vi "test_RxUDPBlockRead.vi"() -> ()   [LabVIEW 2020]
uses:
  <instrlib>/AIM GmbH/_AIM 664/_controls/comm_computedMAC-IP.ctl
  <instrlib>/AIM GmbH/_AIM 664/_controls/comm_verification_rx.ctl
  <instrlib>/AIM GmbH/_AIM 664/_controls/comm_udp_rx.ctl
  <instrlib>/AIM GmbH/_AIM 664/bsp/Controls/ReceiveUDPBlockRead.ctl
  <instrlib>/AIM GmbH/_AIM 664/bsp/Fdx Create Session (Rx-VL-Oriented).vi
  <instrlib>/AIM GmbH/_AIM 664/bsp/Receive/FdxCreateRxVL.vi
  <instrlib>/AIM GmbH/_AIM 664/bsp/Fdx Create UDP Port (RX-CommPort).vi
  <instrlib>/AIM GmbH/_AIM 664/bsp/Fdx Start (Rx).vi
  <instrlib>/AIM GmbH/_AIM 664/bsp/Fdx Stop (Rx).vi
  <instrlib>/AIM GmbH/_AIM 664/AIM664LV.lvlib
panel:
  out "size(s)":i32
  out "RxUDPBlockReadInPortArray":T1[](array[typedef]) {"UDP Handle Out" format="%.0x"; "UDP Handle" format="%.0x"; "Message Buffer" format="%.0x"}
  out "read time uS":u32(graph)
  out "MsgRead Total":u32
  in  "rx fetch rate mS":u32=100
  out "GlobalStat Out":T2={"TotalByteCount"=[139198, 0, 0, 0, 0, 0, 0, 0], "FrameGoodCount"=[1762, 0, 0, 0, 0, 0, 0, 0], "FrameErrorCount"=[0, 0, 0, 0, 0, 0, 0, 0], "BytesPerSecond"=[15800, 0, 0, 0, 0, 0, 0, 0], "FramesPerSecond"=[200, 0, 0, 0, 0, 0, 0, 0], "PhysErrorCount"=[0, 0, 0, 0, 0, 0, 0, 0], "PreamErrorCount"=[0, 0, 0, 0, 0, 0, 0, 0], "UnaligErrorCount"=[0, 0, 0, 0, 0, 0, 0, 0], "CRCErrorCount"=[0, 0, 0, 0, 0, 0, 0, 0], "IFGErrorCount"=[0, 0, 0, 0, 0, 0, 0, 0], "IPErrorCount"=[0, 0, 0, 0, 0, 0, 0, 0], "MACErrorCount"=[0, 0, 0, 0, 0, 0, 0, 0], "NoSfdErrorCount"=[0, 0, 0, 0, 0, 0, 0, 0], "VLLenErrorCount"=[0, 0, 0, 0, 0, 0, 0, 0], "SNIntegrityErrorCount"=[0, 0, 0, 0, 0, 0, 0, 0], "TrafShapingViolationCount"=[0, 0, 0, 0, 0, 0, 0, 0], "MAC1Short"=[0, 0, 0, 0, 0, 0, 0, 0], "MAC64To127Count"=[1762, 0, 0, 0, 0, 0, 0, 0], "MAC128To255Count"=[0, 0, 0, 0, 0, 0, 0, 0], "MAC256To511Count"=[0, 0, 0, 0, 0, 0, 0, 0], "MAC512To1023Count"=[0, 0, 0, 0, 0, 0, 0, 0], "MAC1024To1518Count"=[0, 0, 0, 0, 0, 0, 0, 0], "MACLong"=[0, 0, 0, 0, 0, 0, 0, 0]}
  in  "Control":u32(ring) items=["FDX_RX_GS_RES_NO_CNT", "FDX_RX_GS_RES_ALL_CNT", "FDX_RX_GS_RES_ERR_CNT"]
  out "MsgCount":u32
  out "MsgErrorCount":u32
  out "RxStatus":u32
  out "Info":u32
  in  "stop":bool
  in  "CommPorts":T3[](array[typedef])=[{"PortType"=enum."FDX_UDP_SAMPLING", "SubVIId"=1, "domainID"=1, "sideID"=1, "locationID"=1, "partitionID"=1, "UdpSrcPort"=24, "UdpDstPort"=23, "UdpNumBufMessages"=1, "UdpMaxMessageSize"=512, "UdpSamplingRate"=0}, {"PortType"=enum."FDX_UDP_SAMPLING", "SubVIId"=2, "domainID"=1, "sideID"=1, "locationID"=1, "partitionID"=1, "UdpSrcPort"=34, "UdpDstPort"=33, "UdpNumBufMessages"=1, "UdpMaxMessageSize"=512, "UdpSamplingRate"=0}]
  in  "VL Config":T4={"VlId"=60, "VLRange"=1, "VerificationMode"=0, "Bag"=0, "Jitter"=0, "MaxFrameLength"=0, "MaxSkew"=0, "VLBufSize"=32768, "FilterMode"=0, "FilterPosition"=0, "Padding"=0, "FilterMask"=0, "FilterData"=0, "MinFrameLength"=0} {"FilterMode" items=["FDX_RX_VL_FLT_DIS", "FDX_RX_VL_FLT_ENA ", "FDX_RX_VL_FLT_ENA_INV"]; "VLBufSize" format="%.0x"; "MaxFrameLength" format="%.0x"; "VerificationMode" items=["FDX_RX_VL_CHECK_ENA_DEFAULT"=65535, "FDX_RX_VL_CHECK_REDMAM"=16, "DX_RX_VL_CHECK_TRAFIC"=8, "FDX_RX_VL_CHECK_FRAMESIZE"=4, "FDX_RX_VL_CHECK_SNINTEG"=2, "FDX_RX_VL_CHECK_INVPAC"=1, "FDX_RX_VL_CHECK_DISA"=0]}
  out "computedAddresses":T5={"MACsrc"=[2, 0, 0, 1, 33, 32], "IPsrc"="10.1.33.1", "IPdest"="224.224.0.60"} {"MACsrc" format="%.0x"}
  in  "PortMap":u32=2
  out "PortInitOut":T6={"PortConfig"=0, "PortUsed"=1, "GlobalMemFree"=0, "SharedMemFree"=0} {"PortConfig" items=["FDX_SINGLE", "FDX_REDUNDANT"]}
  in  "port":u32
  in  "board":u32=1
  out "error out":errorcluster
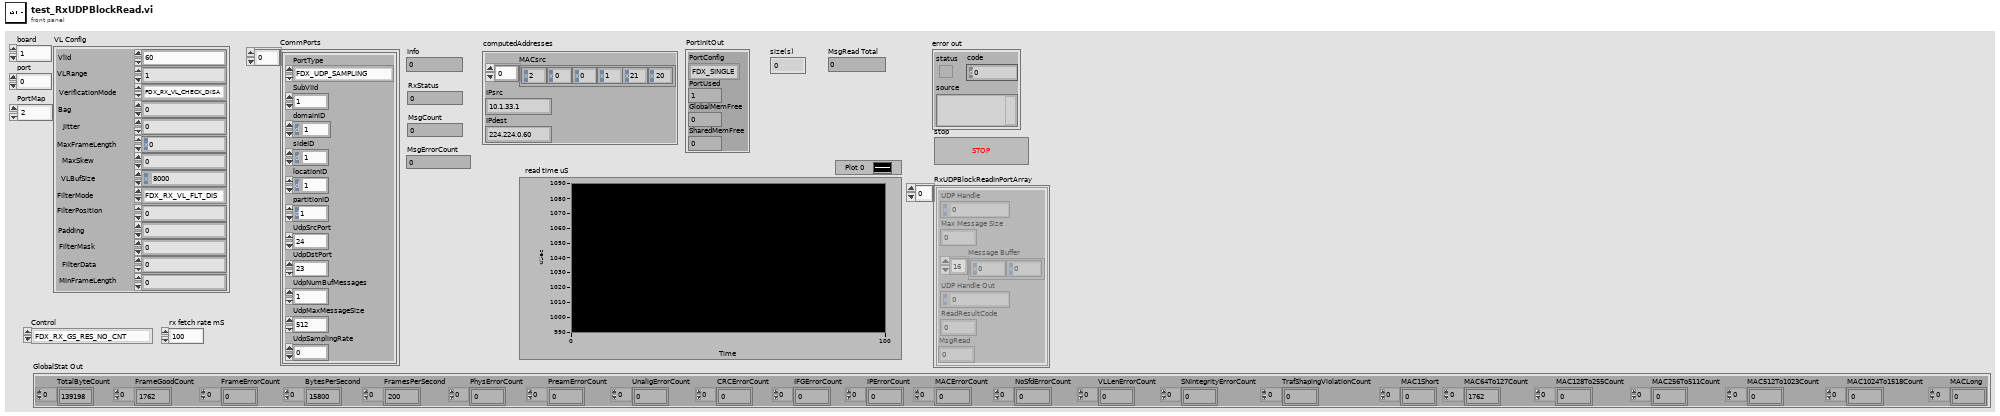
[diagram p1: front panel]
types:
  T1 = typedef "AIM664LV.lvlib/ReceiveUDPBlockRead.ctl" = cluster{"UDP Handle":u32, "Max Message Size":u32, "Message Buffer":u8[], "UDP Handle Out":u32, "ReadResultCode":i32, "MsgRead":u32}
  T2 = cluster{"TotalByteCount":u32[], "FrameGoodCount":u32[], "FrameErrorCount":u32[], "BytesPerSecond":u32[], "FramesPerSecond":u32[], "PhysErrorCount":u32[], "PreamErrorCount":u32[], "UnaligErrorCount":u32[], "CRCErrorCount":u32[], "IFGErrorCount":u32[], "IPErrorCount":u32[], "MACErrorCount":u32[], "NoSfdErrorCount":u32[], "VLLenErrorCount":u32[], "SNIntegrityErrorCount":u32[], "TrafShapingViolationCount":u32[], "MAC1Short":u32[], "MAC64To127Count":u32[], "MAC128To255Count":u32[], "MAC256To511Count":u32[], "MAC512To1023Count":u32[], "MAC1024To1518Count":u32[], "MACLong":u32[]}
  T3 = typedef "AIM664LV.lvlib/comm_udp_rx.ctl" = cluster{"PortType":enum16{"FDX_UDP_SAMPLING", "FDX_UDP_QUEUING"}, "SubVIId":u32, "domainID":u8, "sideID":u8, "locationID":u8, "partitionID":u8, "UdpSrcPort":u16, "UdpDstPort":u16, "UdpNumBufMessages":u32, "UdpMaxMessageSize":u32, "UdpSamplingRate":u32}
  T4 = typedef "AIM664LV.lvlib/comm_verification_rx.ctl" = cluster{"VlId":u16, "VLRange":u32, "VerificationMode":u32, "Bag":u32, "Jitter":u32, "MaxFrameLength":u32, "MaxSkew":u32, "VLBufSize":u32, "FilterMode":u32, "FilterPosition":u32, "Padding":u32, "FilterMask":u32, "FilterData":u32, "MinFrameLength":u32}
  T5 = typedef "AIM664LV.lvlib/comm_computedMAC-IP.ctl" = cluster{"MACsrc":u8[], "IPsrc":string, "IPdest":string}
  T6 = cluster{"PortConfig":u32, "PortUsed":u32, "GlobalMemFree":u32, "SharedMemFree":u32}
  T7 = cluster{"px_UdpBlockReadInPortArray":u64, "px_UdpBlockReadOutPortArray":u64, "size_in":i32, "size_out":i32}
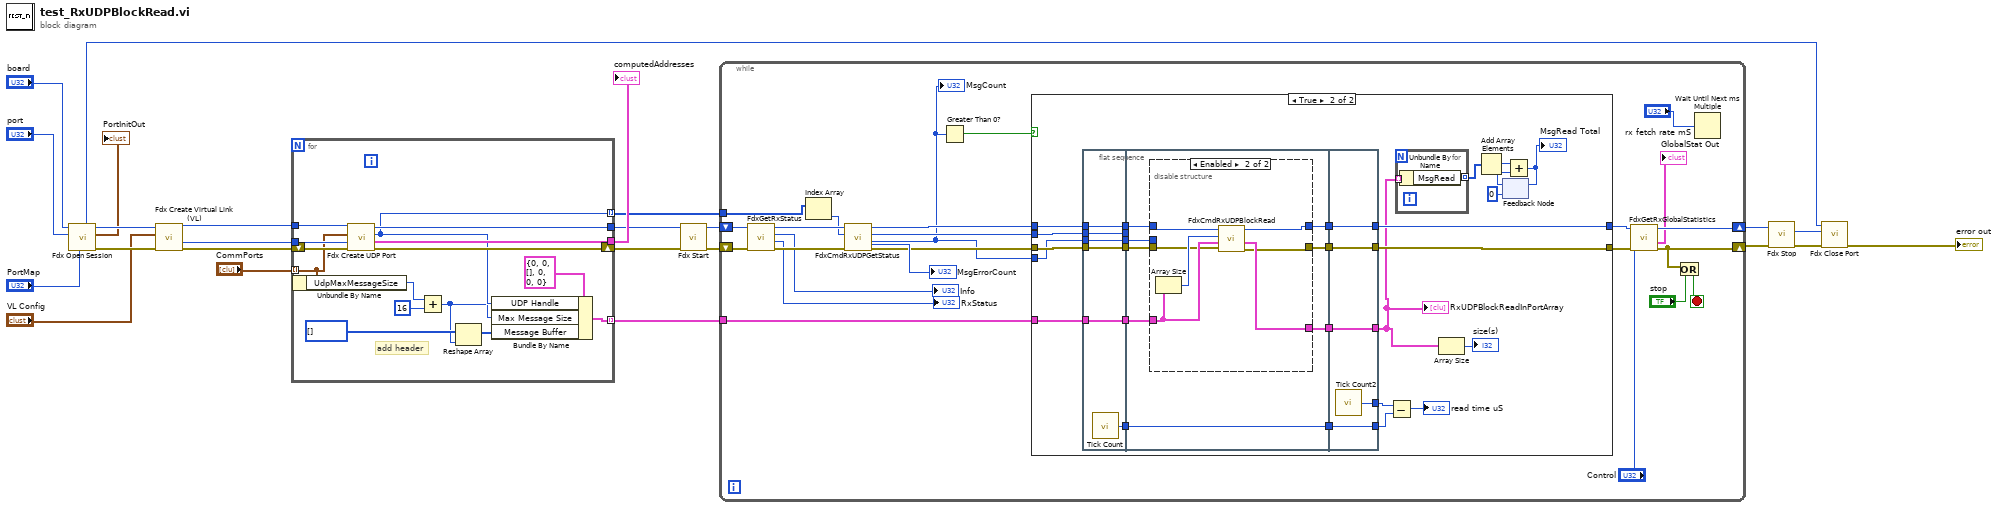
[diagram p0: block diagram]
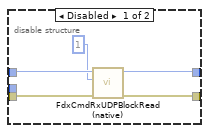
[diagram p3: hidden frame]
diagram:
  n1 = call-poly <instrlib>:"Fdx Open Session.vi"("PortMap"="PortMap", "port"="port", "board"="board") -> ("error out"=w24:errorcluster, "PortInitOut"=→"PortInitOut":T6, "InstrumentHandle_port out"=w20:u32, "InstrumentHandle_board out"=w19:u32)  [unwired: 3 in, 2 out]
  n2 = call-poly <instrlib>:"Fdx Create Virtual Link (VL).vi"("error in (no error)"=w24, "VL Config"="VL Config", "InstrumentHandle_port in"=w20) -> ("error out"=w5:errorcluster, "VlId"=w14:u16, "InstrumentHandle_port out"=w13:u32)  [unwired: 6 in]
  n3 = for {
    tunnel: w14 -> [w38]
    tunnel: w13 -> [w37]
    tunnel: [w36] -> w12
    tunnel: [w35] -> w10
    tunnel: "CommPorts" -> [w30] mode=indexing
    shift-right: [w34] -> w23
    shift-left: w5 -> [w39]
    tunnel: [w31] -> w2 mode=indexing
    tunnel: [w32] -> w1 mode=indexing
    # "add header"
    n4 = Unbundle By Name(w30) -> ("UdpMaxMessageSize"=w27:u32)
    n5 = call-poly <instrlib>:"Fdx Create UDP Port.vi"("error in"=w39, "VlId"=w38, "CommPort Config"=w30, "port handle in"=w37) -> ("error out"=w34:errorcluster, "computedAddresses"=w36:T5, "commPort handle out"=w31:u32, "port handle out"=w35:u32)  [unwired: 4 in]
    n6 = Add(x=w27, y=u32 16) -> (x+y=w26:u32)
    n7 = Reshape Array(u8[] [] ("Message Buffer"), w26) -> (w28:u8[])
    n8 = Bundle By Name(cluster=T1 {"UDP Handle"=0, "Max Message Size"=0, "Message Buffer"=[], "UDP Handle Out"=0, "ReadResultCode"=0, "MsgRead"=0} ("RxUDPBlockReadInPortArray"), "UDP Handle"=w31, "Max Message Size"=w26, "Message Buffer"=w28) -> (w32:T1)
  }
  "computedAddresses" <- w12
  n9 = call-poly <instrlib>:"Fdx Start.vi"("error in"=w23, "InstrumentHandle_port in"=w10) -> ("error out"=w8:errorcluster, "InstrumentHandle_port out"=w9:u32)  [unwired: 8 in]
  n10 = while {
    shift-right: [w44] -> w7
    shift-left: w9 -> [w60]
    shift-right: [w45] -> w6
    shift-left: w8 -> [w59]
    tunnel: w2 -> [w42]
    tunnel: w1 -> [w40]
    stop <- w61 stop-if-true
    n11 = call <instrlib>:"FdxGetRxStatus.vi"("error in"=w59, "InstrumentHandle_port in"=w60) -> ("error out"=w58:errorcluster, "RxStatus"=→"RxStatus":u32, "Info"=→"Info":u32, "InstrumentHandle_port out"=w57:u32)  [unwired: 6 in]
    n12 = Index Array(array=w42) -> (element=w41:u32)  [unwired: 1 in]
    n13 = call <instrlib>:"FdxCmdRxUDPGetStatus.vi"("error in"=w58, "UdpHandle"=w41, "InstrumentHandle_port"=w57) -> ("error out"=w52:errorcluster, "MsgCount"=w49:u32, "UdpHandle Out"=w51:u32, "InstrumentHandle_port"=w50:u32, "MsgErrorCount"=→"MsgErrorCount":u32)  [unwired: 4 in]
    "MsgCount" <- w49
    n14 = Greater Than 0?(x=w49) -> (x > 0?=w53:bool)
    n15 = case shown="True" w53 {
      tunnel: w52 -> [w64 w90]
      tunnel: w51 -> [_ w92]
      tunnel: w50 -> [w65 w91]
      tunnel: [w65 w87] -> w47
      tunnel: [w64 w88] -> w48
      tunnel: w49 -> [_ w89]
      tunnel: w40 -> [_ w71]
      frame False {
      }
      frame True {
        n16 = flat-sequence {
          tunnel: w89 -> [w97]
          tunnel: w90 -> [w98]
          tunnel: w91 -> [w99]
          tunnel: w92 -> [w100]
          tunnel: [w100] -> w83
          tunnel: [w99] -> w82
          tunnel: [w98] -> w81
          tunnel: [w97] -> w80
          tunnel: [w96] -> w74
          tunnel: [w95] -> w72
          tunnel: w71 -> [w95]
          tunnel: w83 -> [_]
          tunnel: w82 -> [w108]
          tunnel: w81 -> [w107]
          tunnel: w80 -> [w106]
          tunnel: [w105] -> w79
          tunnel: [w104] -> w78
          tunnel: [w103] -> w75
          tunnel: w74 -> [w103]
          tunnel: w72 -> [w102]
          tunnel: [w101] -> w70
          tunnel: [w125] -> w87
          tunnel: [w126] -> w88
          tunnel: w79 -> [w126]
          tunnel: w78 -> [w125]
          tunnel: [w124] -> w77
          tunnel: [w123] -> w76
          tunnel: w75 -> [w123]
          tunnel: [w122] -> w67
          tunnel: w70 -> [w122]
          frame #0 {
            n17 = call "Tick Count"() -> ("Tick Count(uSec)"=w96:u32)
          }
          frame #1 {
            n18 = disable-structure shown="Enabled" {
              disable-tunnel: w108 -> [w113 w121]
              disable-tunnel: w107 -> [w112 w118]
              disable-tunnel: w106 -> [_ _]
              disable-tunnel: [w111 w115] -> w105
              disable-tunnel: [w110 w117] -> w104
              disable-tunnel: w102 -> [_ w120]
              disable-tunnel: [_ w116] -> w101
              frame Disabled {
                n19 = call "FdxCmdRxUDPBlockRead(native).vi"("error in"=w112, "PortCountIn"=u32 1, "InstrumentHandle_port"=w113) -> ("error out"=w111:errorcluster, "InstrumentHandle_port"=w110:u32, "ubrx in"=w114:T7)  [unwired: 5 in, 1 out]
              }
              frame Enabled {
                n20 = Array Size(array=w120) -> (size(s)=w119:i32)
                n21 = call <instrlib>:"FdxCmdRxUDPBlockRead.vi"("error in"=w118, "RxUDPBlockReadInPortArray"=w120, "PortCountIn"=w119, "InstrumentHandle_port"=w121) -> ("error out"=w115:errorcluster, "RxUDPBlockReadInPortArray"=w116:T1[], "InstrumentHandle_port"=w117:u32)  [unwired: 5 in]
              }
            }
          }
          frame #2 {
            n22 = call "Tick Count2"() -> ("Tick Count(uSec)"=w124:u32)
          }
        }
        n23 = Subtract(x=w77, y=w76) -> (x-y=→"read time uS":u32)
        n24 = for {
          tunnel: w67 -> [w94] mode=indexing
          tunnel: [w93] -> w69 mode=indexing
          n25 = Unbundle By Name(w94) -> ("MsgRead"=w93:u32)
        }
        n26 = Array Size(array=w67) -> (size(s)=→"size(s)":i32)
        n27 = Add Array Elements(numeric array=w69) -> (sum=w68:u32)
        n28 = feedback #1(u32 0 ("MsgRead")) -> (w85:u32)
        n29 = Add(x=w68, y=w85) -> (x+y=w84:u32)
        "MsgRead Total" <- w84
        n30 = feedback-in #1(w84) -> ()
        "RxUDPBlockReadInPortArray" <- w67
      }
    }
    n31 = call <instrlib>:"FdxGetRxGlobalStatistics.vi"("error in"=w48, "Control"="Control", "InstrumentHandle_port in"=w47) -> ("error out"=w45:errorcluster, "GlobalStat Out"=→"GlobalStat Out":T2, "InstrumentHandle_port out"=w44:u32)  [unwired: 6 in]
    n32 = Or(x=w45, y="stop") -> (x .or. y?=w61:bool)
    n33 = Wait Until Next ms Multiple(millisecond multiple="rx fetch rate mS") -> ()  [unwired: 1 out]
  }
  n34 = call-poly <instrlib>:"Fdx Stop.vi"("error in"=w6, "InstrumentHandle_port in"=w7) -> ("error out"=w22:errorcluster, "InstrumentHandle_port out"=w21:u32)  [unwired: 8 in]
  n35 = call <instrlib>:"Fdx Close Port.vi"("error in"=w22, "InstrumentHandle_port in"=w21, "InstrumentHandle_board in"=w19) -> ("error out"=→"error out":errorcluster)  [unwired: 7 in, 1 out]
